vi "Make Unique Movement Proposals.vi"(0 "Elves in":T2(c390)) -> (1 "Elves' Movement Proposals":map{T1, T1}(c390), 2 "Elves out":T2(c390))   [LabVIEW 2020, in "AoC 2022.lvlib"]
uses:
  AoC 2022.lvlib
  Day 15 - Beacon Exclusion Zone/private/Location.ctl
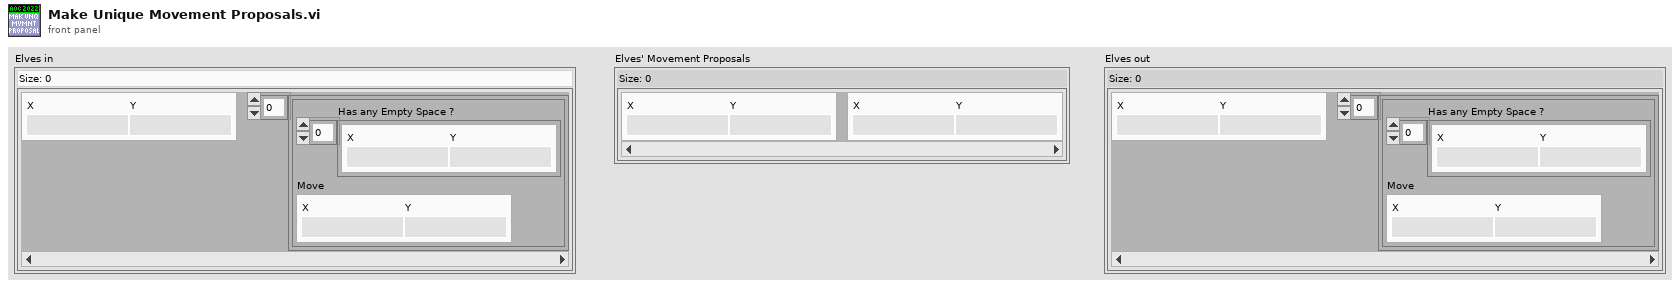
[diagram p1: front panel]
types:
  T1 = typedef "AoC 2022.lvlib/Location.ctl" = cluster{"X":i32, "Y":i32}
  T2 = map{T1, cluster{"Has any Empty Space ?":T1[], "Move":T1}[]}
  T3 = cluster{"Has any Empty Space ?":T1[], "Move":T1}[]
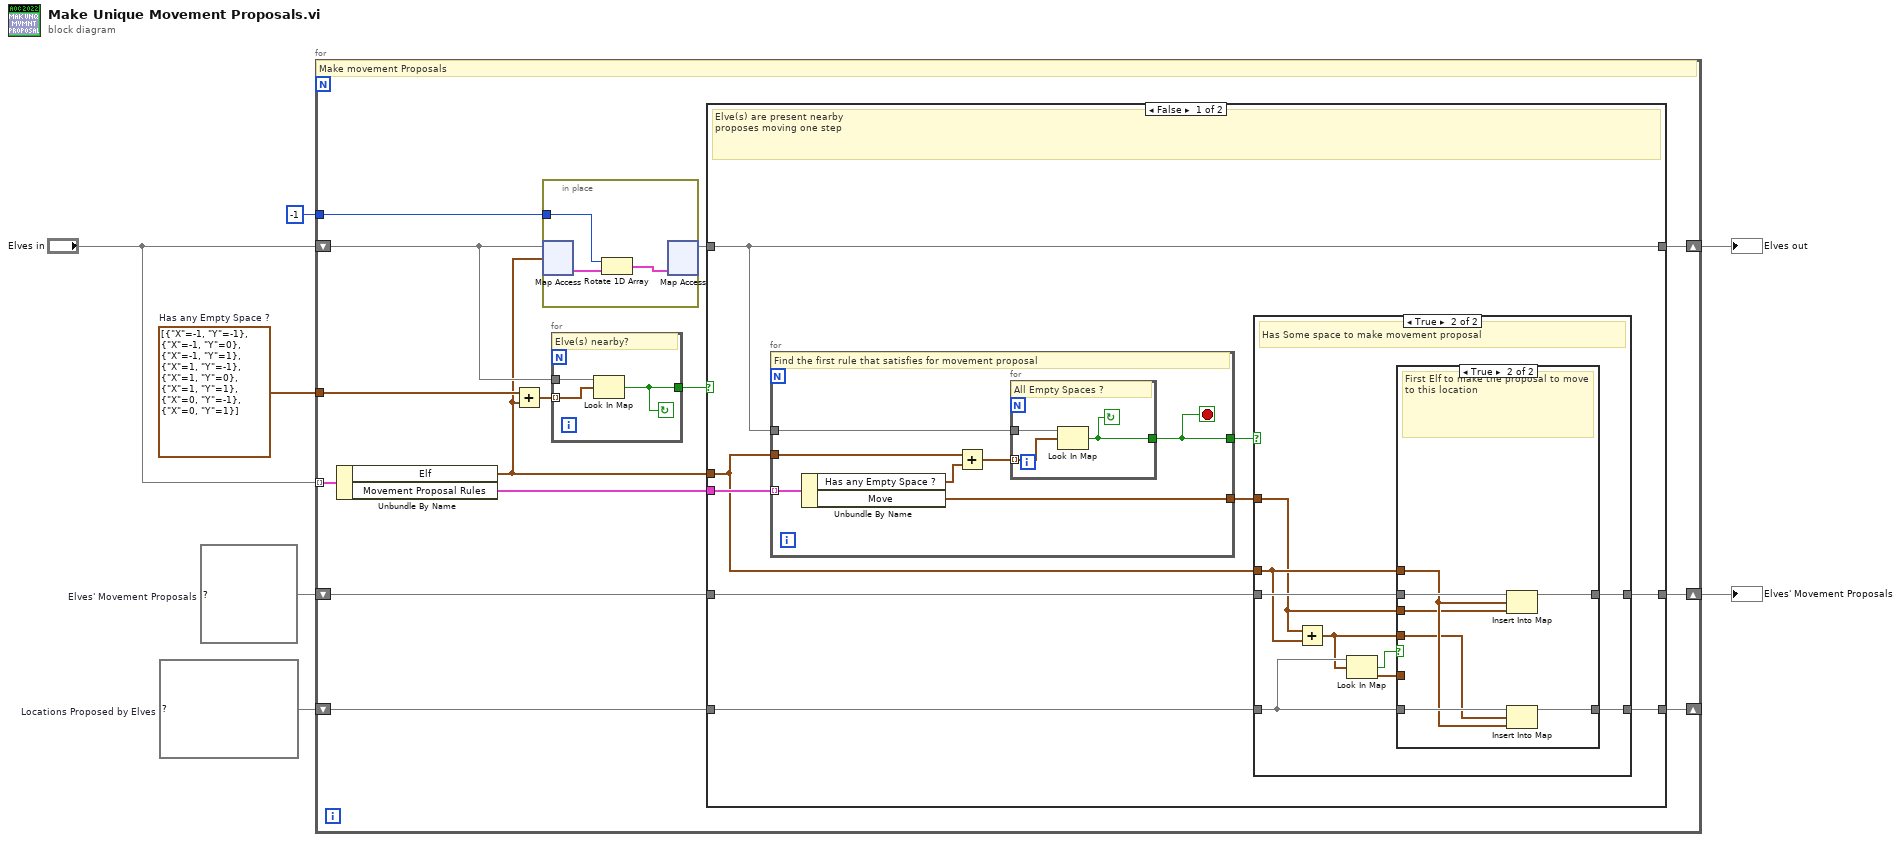
[diagram p0: block diagram]
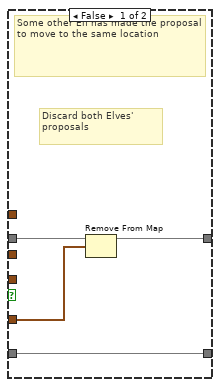
[diagram p3: hidden frame]
diagram:
  w5 = map{T1, T1} {}  # Locations Proposed by Elves
  w4 = map{T1, T1} {}  # Elves' Movement Proposals
  w3 = T1[] [{"X"=-1, "Y"=-1}, {"X"=-1, "Y"=0}, {"X"=-1, "Y"=1}, {"X"=1, "Y"=-1}, {"X"=1, "Y"=0}, {"X"=1, "Y"=1}, {"X"=0, "Y"=-1}, {"X"=0, "Y"=1}]  # Has any Empty Space ?
  n1 = for {
    tunnel: "Elves in" -> [w21] mode=indexing
    shift-right: [w20] -> w7
    shift-left: "Elves in" -> [w11]
    tunnel: -1 -> [w9]
    tunnel: w3 -> [w19]
    shift-right: [w15] -> _
    shift-left: w5 -> [w14]
    shift-right: [w13] -> w6
    shift-left: w4 -> [w12]
    # "Make movement Proposals"
    n2 = Unbundle By Name(w21) -> ("Elf"=w8:T1, "Movement Proposal Rules"=w16:T3)
    n3 = Add(x=w19, y=w8) -> (x+y=w18:T1[])
    n4 = in-place {
      in-place-border: w9 -> [w25]
      n5 = in-place-map #1(w11, w8) -> (w27:T3)  [unwired: 1 in, 1 out]
      n6 = Rotate 1D Array(1:w27, 2:w25) -> (0:w26:T3)
      n7 = in-place-map #1(w26) -> (w10:T2)  [unwired: 1 in, 2 out]
    }
    n8 = for {
      tunnel: w18 -> [w23] mode=indexing
      tunnel: w11 -> [w24]
      tunnel: [w22] -> w17
      stop <- w22 continue-if-true
      # "Elve(s) nearby?"
      n9 = Look In Map(map=w24, key=w23) -> (key not found?=w22:bool)  [unwired: 1 in, 1 out]
    }
    n10 = case shown="False" w17 {
      tunnel: w10 -> [w28 w69]
      tunnel: [w28 w69] -> w20
      tunnel: w16 -> [w36 _]
      tunnel: [w31 w71] -> w15
      tunnel: w14 -> [w33 w71]
      tunnel: [w32 w70] -> w13
      tunnel: w12 -> [w34 w70]
      tunnel: w8 -> [w29 _]
      frame False {
        # "Elve(s) are present nearby\nproposes moving one step"
        n11 = for {
          tunnel: w36 -> [w65] mode=indexing
          tunnel: w29 -> [w63]
          tunnel: w28 -> [w62]
          tunnel: [w60] -> w35
          tunnel: [w59] -> w30
          stop <- w60 stop-if-true
          # "Find the first rule that satisfies for movement proposal"
          n12 = Unbundle By Name(w65) -> ("Has any Empty Space ?"=w64:T1[], "Move"=w59:T1)
          n13 = Add(x=w63, y=w64) -> (x+y=w61:T1[])
          n14 = for {
            tunnel: w62 -> [w68]
            tunnel: w61 -> [w67] mode=indexing
            tunnel: [w66] -> w60
            stop <- w66 continue-if-true
            # "All Empty Spaces ?"
            n15 = Look In Map(map=w68, key=w67) -> (key not found?=w66:bool)  [unwired: 1 in, 1 out]
          }
        }
        n16 = case shown="True" w35 {
          tunnel: w34 -> [w38 w46]
          tunnel: w33 -> [w37 w43]
          tunnel: [w38 w47] -> w32
          tunnel: [w37 w45] -> w31
          tunnel: w30 -> [_ w40]
          tunnel: w29 -> [_ w41]
          frame False {
            # "No Valid Directions to propose for movement"
          }
          frame True {
            # "Has Some space to make movement proposal"
            n17 = Add(x=w40, y=w41) -> (x+y=w39:T1)
            n18 = Look In Map(map=w43, key=w39) -> (key not found?=w44:bool, value=w42:T1)  [unwired: 1 in]
            n19 = case shown="True" w44 {
              tunnel: w43 -> [w51 w56]
              tunnel: [w50 w57] -> w47
              tunnel: w46 -> [w49 w58]
              tunnel: [w51 w55] -> w45
              tunnel: w41 -> [_ w54]
              tunnel: w40 -> [_ w53]
              tunnel: w42 -> [w48 _]
              tunnel: w39 -> [_ w52]
              frame False {
                # "Discard both Elves' proposals"
                # "Some other Elf has made the proposal to move to the same location"
                n20 = Remove From Map(10:w48, 11:w49) -> (3:w50:map{T1, T1})  [unwired: 2 out]
              }
              frame True {
                # "First Elf to make the proposal to move to this location"
                n21 = Insert Into Map(map in=w58, key=w54, value=w53) -> (map out=w57:map{T1, T1})  [unwired: 2 out]
                n22 = Insert Into Map(map in=w56, key=w52, value=w54) -> (map out=w55:map{T1, T1})  [unwired: 2 out]
              }
            }
          }
        }
      }
      frame True {
        # "No Elves are present nearby\ndoes not do anything"
      }
    }
  }
  "Elves out" <- w7
  "Elves' Movement Proposals" <- w6
